vi "createOutputFile.vi"(10 "name or relative path":string, 11 "Data TIFF File":path) -> (3 "new tiff pointer":i64)   [LabVIEW 2013]
uses:
  imagereconstruction/x64/Release/labviewdll.dll
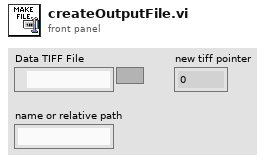
[diagram p1: front panel]
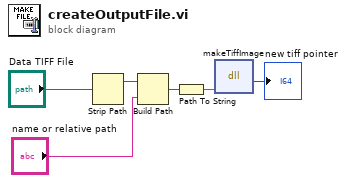
[diagram p0: block diagram]
diagram:
  n1 = Strip Path(path="Data TIFF File") -> (stripped path=w1:path)  [unwired: 1 out]
  n2 = Build Path(base path=w1, name or relative path="name or relative path") -> (appended path=w2:path)
  n3 = Path To String(path=w2) -> (string=w4:string)
  n4 = dll-call lib="D:/work/uni/FYP/reconrepo/imagereconstruction/x64/Release/labviewdll.dll" fn="makeTiffImage"("resultPath"=w4) -> ("return type"=→"new tiff pointer":i64)  [unwired: 4 in, 2 out]
